vi "Current EXE File Path.vi"(8 "error in (no error)":errorcluster) -> (0 "error out":errorcluster, 3 "Current EXE Path":path)   [LabVIEW 2014, in "SLL Application.lvlib"]
doc: "Provides the current EXE file path. \n\nThis will not work in LabVIEW development environment."
uses:
  SLL Application.lvlib
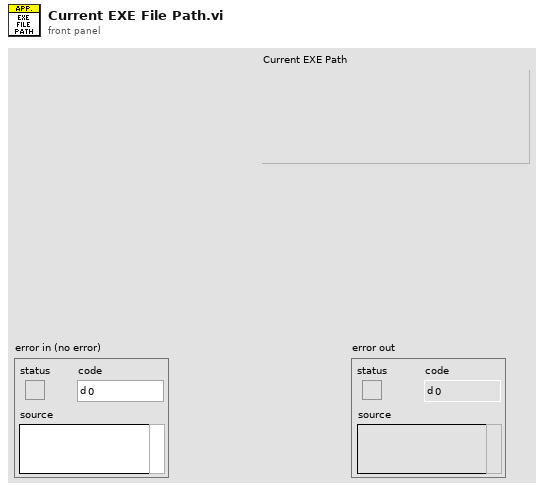
[diagram p1: front panel]
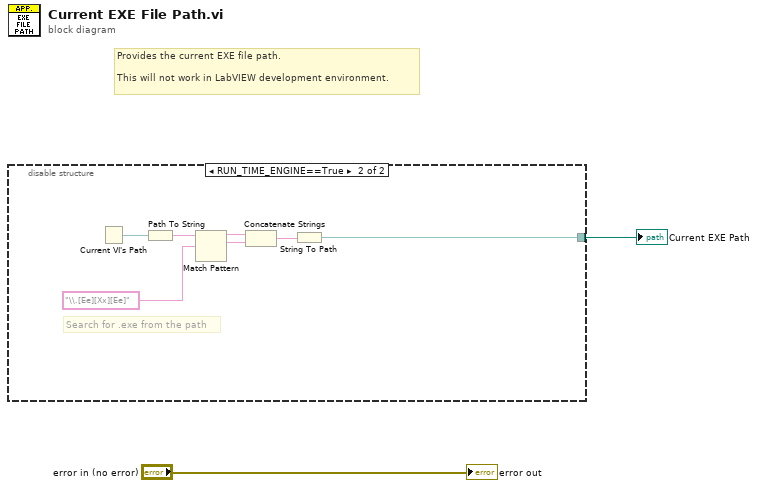
[diagram p0: block diagram]
diagram:
  # "Provides the current EXE file path. \n\nThis will not work in LabVIEW development environment."
  n1 = disable-structure shown="RUN_TIME_ENGINE==True" {
    disable-tunnel: [_ w3] -> w1
    frame condition #0 (active) {
    }
    frame condition #1 {
      # "Search for .exe from the path"
      n2 = Current VI's Path() -> (path=w4:path)
      n3 = Path To String(path=w4) -> (string=w9:string)
      n4 = Match Pattern(string=w9, regular expression="\\.[Ee][Xx][Ee]") -> (before substring=w6:string, match substring=w7:string)  [unwired: 1 in, 2 out]
      n5 = Concatenate Strings(w6, w7) -> (w8:string)
      n6 = String To Path(string=w8) -> (path=w3:path)
    }
  }
  "Current EXE Path" <- w1
  "error out" <- "error in (no error)"
